vi "can_readStatus.vi"(8 "error in (no error)":errorcluster, 11 "Instrument in":refnum<class "Instrument.lvclass">) -> (0 "error out":errorcluster, 1 "fault":u8[](array[numeric]), 2 "Status":u16[](array[numeric]), 3 "Instrument out":refnum<class "Instrument.lvclass">, 4 "temperature":sgl[](array[numeric]))   [LabVIEW 2019, in "Instrument.lvclass"]
uses:
  Instrument.lvclass
  Instrument.lvclass/Instrument.ctl
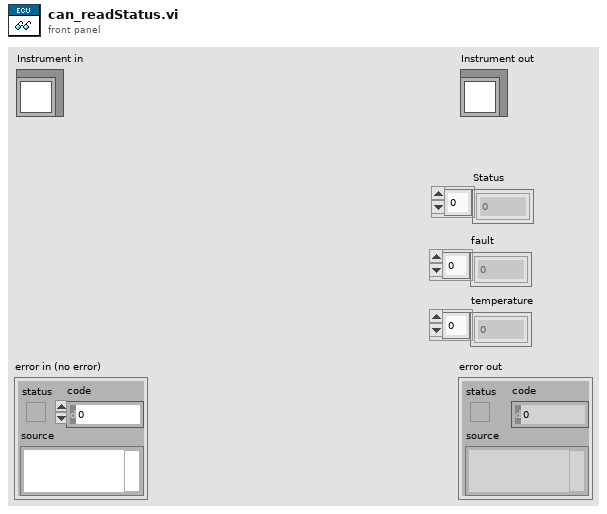
[diagram p1: front panel]
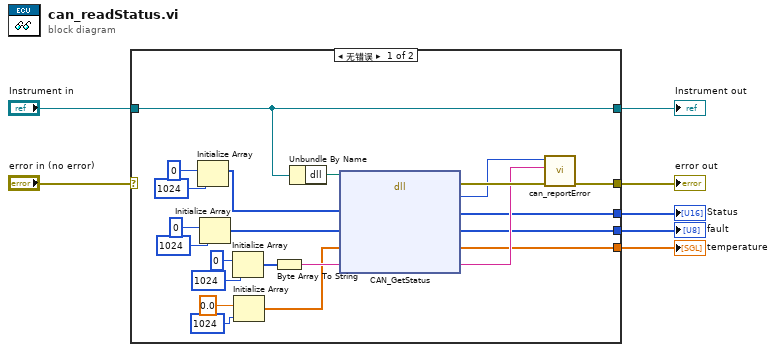
[diagram p0: block diagram]
diagram:
  n1 = case shown="无错误" "error in (no error)" {
    selector: "error in (no error)" -> [_ w31]
    tunnel: [w24 w31] -> w6
    tunnel: [w29 w30] -> w4
    tunnel: "Instrument in" -> [w29 w30]
    tunnel: [w19 _] -> w3
    tunnel: [w18 _] -> w2
    tunnel: [w17 _] -> w1
    frame No Error {
      n2 = Initialize Array(u16 0 ("element"), 1024 ("dimension size")) -> (w11:u16[])
      n3 = Initialize Array(u8 0 ("element"), 1024 ("dimension size")) -> (w14:u8[])
      n4 = Initialize Array(u8 0 ("element"), 1024 ("dimension size")) -> (w21:u8[])
      n5 = Initialize Array(sgl 0.0 ("element"), 1024 ("dimension size")) -> (w8:sgl[])
      n6 = Byte Array To String(unsigned byte array=w21) -> (string=w20:string)
      n7 = Unbundle By Name(w29) -> ("dll"=w28:path)
      n8 = dll-call lib="C:/Dev/22KW-Dyno/software/data/DynoAPI.dll" fn="CAN_GetStatus"(path in=w28, "status"=w11, "fault"=w14, "temperature"=w8, "ErrorMsg"=w20) -> (error out=w27:errorcluster, "return type"=w26:i32, "status"=w19:u16[], "fault"=w18:u8[], "temperature"=w17:sgl[], "ErrorMsg"=w25:string)  [unwired: 2 in, 1 out]
      n9 = call "can_reportError.vi"("error in (no error)"=w27, "errorMsg"=w25, "return type"=w26) -> ("error out"=w24:errorcluster)  [unwired: 8 in]
    }
    frame Error {
    }
  }
  "error out" <- w6
  "Instrument out" <- w4
  "temperature" <- w1
  "fault" <- w2
  "Status" <- w3
